vi "SetEndDate.vi"(8 "error in":errorcluster, 10 "EndDate":timestamp, 11 "SequenceRun in":refnum<class "SequenceRun.lvclass">) -> (0 "error out":errorcluster, 3 "SequenceRun out":refnum<class "SequenceRun.lvclass">)   [LabVIEW 2021, in "ProligentXMLGenerator.lvlib" / "SequenceRun.lvclass"]
doc: "Defines the actual date where the sequence run ended.\nIf 'SequenceExecutionStatus' is equal to 'NOT_COMPLETED' this value must be ommited.\nSequenceRunId must have been provided to allow sequence run updates through DIT increment.\nThis value must be greater or equal than StartDate.\n\nNote that the if the Data Warehouse already contains this sequence run but it is not already\nclosed, the EndDate written in the Data Warehouse will be set according to the following rule: EndDate(in database) = StartDate(in database) + (EndDate(from xml) - StartDate(from xml)).\n\nThis value is restricted to \"1900-01-01T00:00:00Z\" -\"2100-01-01T00:00:00Z\"."
uses:
  SequenceRun.lvclass
  SequenceRun.lvclass/SequenceRun.ctl
  Base/DateTime/DateTime.lvclass
  Base/ExecutionStatus/Value.ctl
  Base/ExecutionStatus/ExecutionStatus.lvclass
  Base/Attribute/Attribute.lvclass
  C:/Projects/proligent-xml-generator-labview/src/ProligentXMLGenerator/Base/Attribute/Attribute.lvclass
  C:/Projects/proligent-xml-generator-labview/src/ProligentXMLGenerator/Base/DateTime/DateTime.lvclass
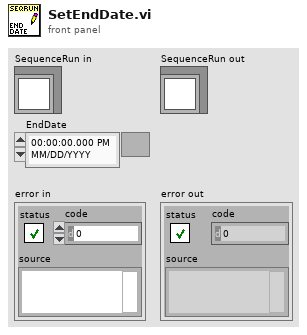
[diagram p1: front panel]
types:
  T1 = typedef "ProligentXMLGenerator.lvlib/ExecutionStatus.lvclass/Value.ctl" = enum16{"PASS", "FAIL", "NOT_COMPLETED", "ABORTED"}
  T2 = typedef "ProligentXMLGenerator.lvlib/SequenceRun.lvclass/Data.ctl" = cluster{"Name":string, "StepRuns":refnum<class "StepRun.lvclass">[], "Characteristics":refnum<class "Characteristic.lvclass">[], "Documents":refnum<class "Document.lvclass">[], "FailureReferences":refnum<class "FailureReference.lvclass">[], "CustomData":refnum<class "CustomData.lvclass">, "StartDate":refnum<class "DateTime.lvclass">, "EndDate":refnum<class "DateTime.lvclass">, "SequenceExecutionStatus":refnum<class "ExecutionStatus.lvclass">, "SequenceRunId":refnum<class "Guid.lvclass">, "SequenceFullName":refnum<class "SequenceFullName.lvclass">, "SequenceVersion":refnum<class "NonEmptyString_64.lvclass">, "StationFullName":refnum<class "FullName.lvclass">, "User":refnum<class "NonEmptyString_255.lvclass">, "TimeZoneInfoId":string}
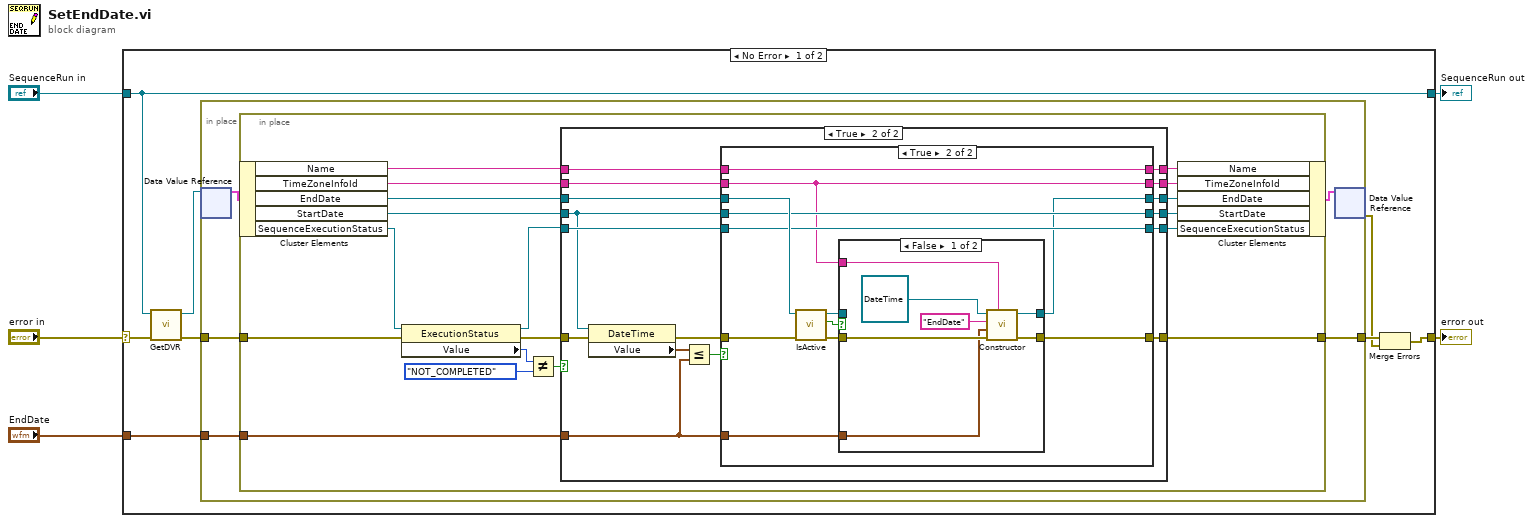
[diagram p0: block diagram]
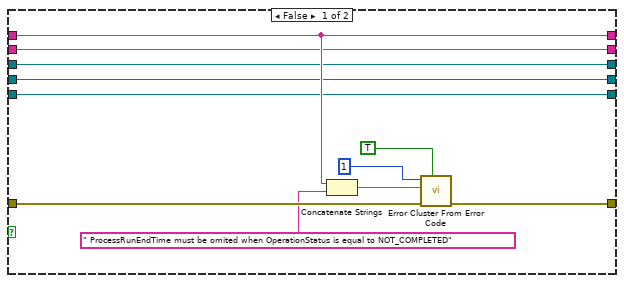
[diagram p2: hidden frame]
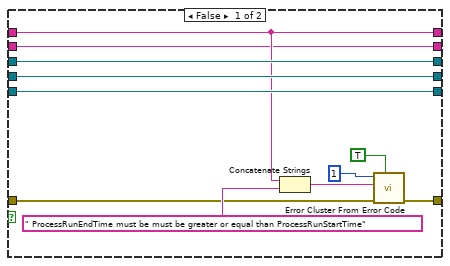
[diagram p3: hidden frame]
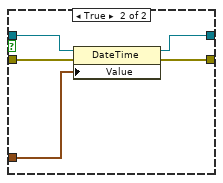
[diagram p4: hidden frame]
diagram:
  n1 = case shown="No Error" "error in" {
    selector: "error in" -> [w12 w99]
    tunnel: "SequenceRun in" -> [w7 w100]
    tunnel: [w9 w99] -> w3
    tunnel: "EndDate" -> [w8 _]
    tunnel: [w7 w100] -> w1
    frame No Error {
      n2 = call "GetDVR.vi"("error in"=w12, "SequenceRun"=w7) -> ("error out"=w11:errorcluster, "DVRReference"=w13:refnum<data-value>)  [unwired: 8 in]
      n3 = in-place "In Place Element Structure" {
        in-place-border: w11 -> [w16]
        in-place-border: [w18] -> w10
        in-place-border: w8 -> [w17]
        n4 = in-place-dvr #1(w13) -> (w15:T2)  [unwired: 1 out]
        n5 = in-place "In Place Element Structure" {
          in-place-border: [w36] -> w18
          in-place-border: w17 -> [w35]
          in-place-border: w16 -> [w34]
          n6 = in-place-cluster #2(w15) -> ("Name"=w26:string, "TimeZoneInfoId"=w19:string, "EndDate"=w27:refnum<class "DateTime.lvclass">, "StartDate"=w28:refnum<class "DateTime.lvclass">, "SequenceExecutionStatus"=w29:refnum<class "ExecutionStatus.lvclass">)
          n7 = property on="Property Node" class="ExecutionStatus"(reference=w29, error in=w34) -> (reference out=w25:refnum<class "ExecutionStatus.lvclass">, error out=w33:errorcluster, "Value"=w32:T1)
          n8 = Not Equal?(x=w32, y=Value."NOT_COMPLETED") -> (x != y?=w30:bool)
          n9 = case shown="True" w30 {
            tunnel: [w43 w63] -> w36
            tunnel: w35 -> [_ w58]
            tunnel: w27 -> [w40 w62]
            tunnel: w33 -> [w44 w61]
            tunnel: w26 -> [w41 w56]
            tunnel: w28 -> [w39 w52]
            tunnel: w25 -> [w38 w55]
            tunnel: [w38 w54] -> w24
            tunnel: [w40 w53] -> w23
            tunnel: [w39 w51] -> w22
            tunnel: [w41 w50] -> w21
            tunnel: [w37 w49] -> w20
            tunnel: w19 -> [w37 w48]
            frame False {
              n10 = Concatenate Strings(w41, " ProcessRunEndTime must be omited when OperationStatus is equal to NOT_COMPLETED" ("string")) -> (w45:string)
              n11 = call <vilib>:"Error Cluster From Error Code.vi"("show call chain? (False)"=TRUE, "error in (no error)"=w44, "error message (\"\")"=w45, "error code (0)"=1) -> ("error out"=w43:errorcluster)  [unwired: 5 in]
            }
            frame True {
              n12 = property on="Property Node" class="DateTime"(reference=w52, error in=w61) -> (error out=w60:errorcluster, "Value"=w59:timestamp)  [unwired: 1 out]
              n13 = Less Or Equal?(x=w59, y=w58) -> (x <= y?=w57:bool)
              n14 = case shown="True" w57 {
                tunnel: [w69 w86] -> w63
                tunnel: w62 -> [w67 w84]
                tunnel: w60 -> [w70 w82]
                tunnel: w58 -> [_ w81]
                tunnel: w56 -> [w65 w76]
                tunnel: w55 -> [w68 w79]
                tunnel: [w68 w79] -> w54
                tunnel: [w67 w77] -> w53
                tunnel: w52 -> [w66 w78]
                tunnel: [w66 w78] -> w51
                tunnel: [w65 w76] -> w50
                tunnel: [w64 w75] -> w49
                tunnel: w48 -> [w64 w75]
                frame False {
                  n15 = Concatenate Strings(w65, " ProcessRunEndTime must be must be greater or equal than ProcessRunStartTime" ("string")) -> (w72:string)
                  n16 = call <vilib>:"Error Cluster From Error Code.vi"("show call chain? (False)"=TRUE, "error in (no error)"=w70, "error message (\"\")"=w72, "error code (0)"=1) -> ("error out"=w69:errorcluster)  [unwired: 5 in]
                }
                frame True {
                  n17 = call "IsActive.vi"("error in"=w82, "Attribute in"=w84) -> ("error out"=w85:errorcluster, "IsActive"=w80:bool, "Attribute in"=w83:refnum<class "DateTime.lvclass">)  [unwired: 7 in]
                  n18 = case shown="False" w80 {
                    tunnel: [w92 w98] -> w86
                    tunnel: w81 -> [w89 w97]
                    tunnel: w85 -> [w93 w96]
                    tunnel: w83 -> [_ w95]
                    tunnel: [w88 w94] -> w77
                    tunnel: w75 -> [w87 _]
                    frame False {
                      n19 = call-dynamic "Constructor.vi"("TimeZoneInfoId"=w87, "error in"=w93, "Value"=w89, "Name"="EndDate", "DateTime in"=refnum<class "DateTime.lvclass"> refnum ("ProligentResultProcessor:DateTime")) -> ("error out"=w92:errorcluster, "DateTime out"=w88:refnum<class "DateTime.lvclass">)  [unwired: 5 in]
                    }
                    frame True {
                      n20 = property on="Property Node" class="DateTime"(reference=w95, error in=w96, "Value"=w97) -> (reference out=w94:refnum<class "DateTime.lvclass">, error out=w98:errorcluster)
                    }
                  }
                }
              }
            }
          }
          n21 = in-place-cluster #2("Name"=w21, "TimeZoneInfoId"=w20, "EndDate"=w23, "StartDate"=w22, "SequenceExecutionStatus"=w24) -> (w14:T2)
        }
        n22 = in-place-dvr #1(w14) -> (w6:errorcluster)  [unwired: 1 out]
      }
      n23 = Merge Errors(w10, w6) -> (w9:errorcluster)
    }
    frame Error {
    }
  }
  "error out" <- w3
  "SequenceRun out" <- w1
